vi "Make File Tree.vi"(8 "Error In":errorcluster, 10 "TreeControl in":refnum<vi>, 11 "WAD Main Cluster":T1) -> (0 "Error Out":errorcluster, 2 "TreeControl OUT":refnum<vi>, 3 "WAD Main Cluster OUT":T1)   [LabVIEW 2017]
uses:
  WAD_MainCluster.ctl
  TextureList.ctl
  PatchList.ctl
  Lumps.ctl
  <userlib>/_OpenG.lib/array/array.llb/Filter 1D Array (String)__ogtk.vi
  <vilib>/regexp/Match Regular Expression.xnode
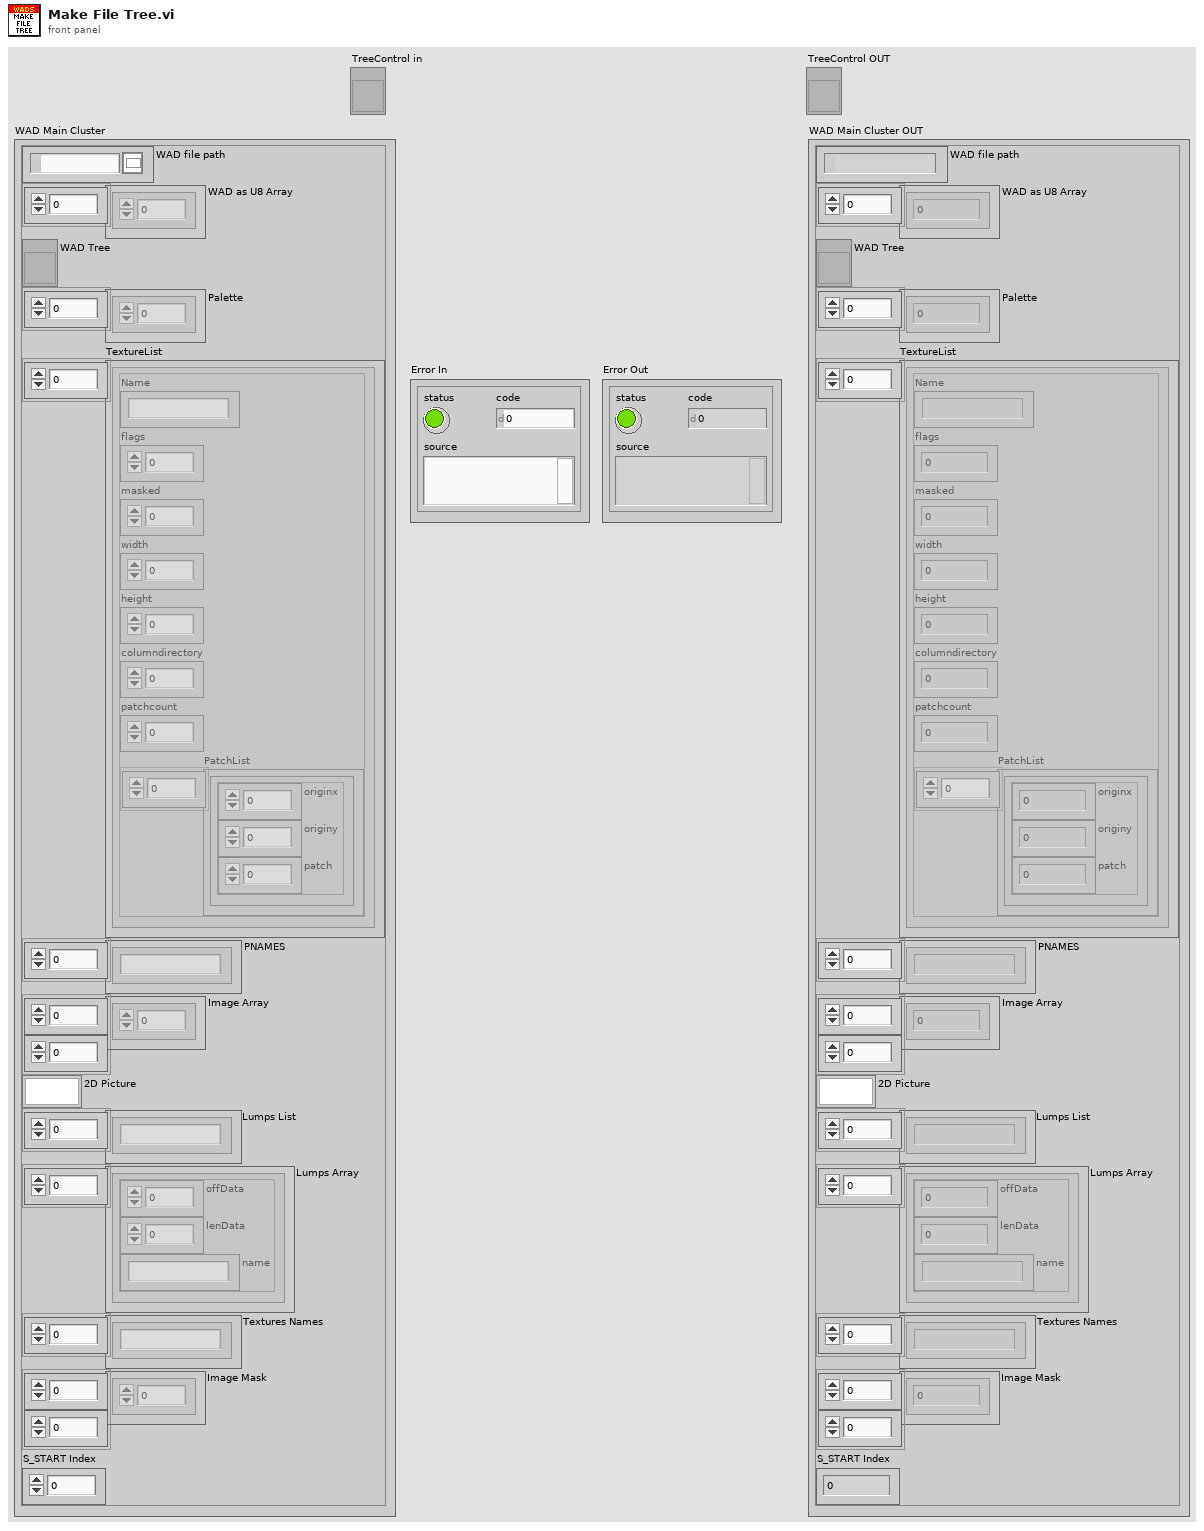
[diagram p1: front panel]
types:
  T1 = typedef "WAD_MainCluster.ctl" = cluster{"WAD file path":path, "WAD as U8 Array":u8[], "WAD Tree":refnum<vi>, "Palette":u32[], "TextureList":T2[], "PNAMES":string[], "Image Array":i16[][], "2D Picture":picture, "Lumps List":string[], "Lumps Array":T4[], "Textures Names":string[], "Image Mask":i16[][], "S_START Index":i32}
  T2 = typedef "TextureList.ctl" = cluster{"Name":string, "flags":u16, "masked":i16, "width":i16, "height":i16, "columndirectory":u32, "patchcount":i16, "PatchList":T3[]}
  T3 = typedef "PatchList.ctl" = cluster{"originx":i16, "originy":i16, "patch":i16}
  T4 = typedef "Lumps.ctl" = cluster{"offData":i32, "lenData":i32, "name":string}
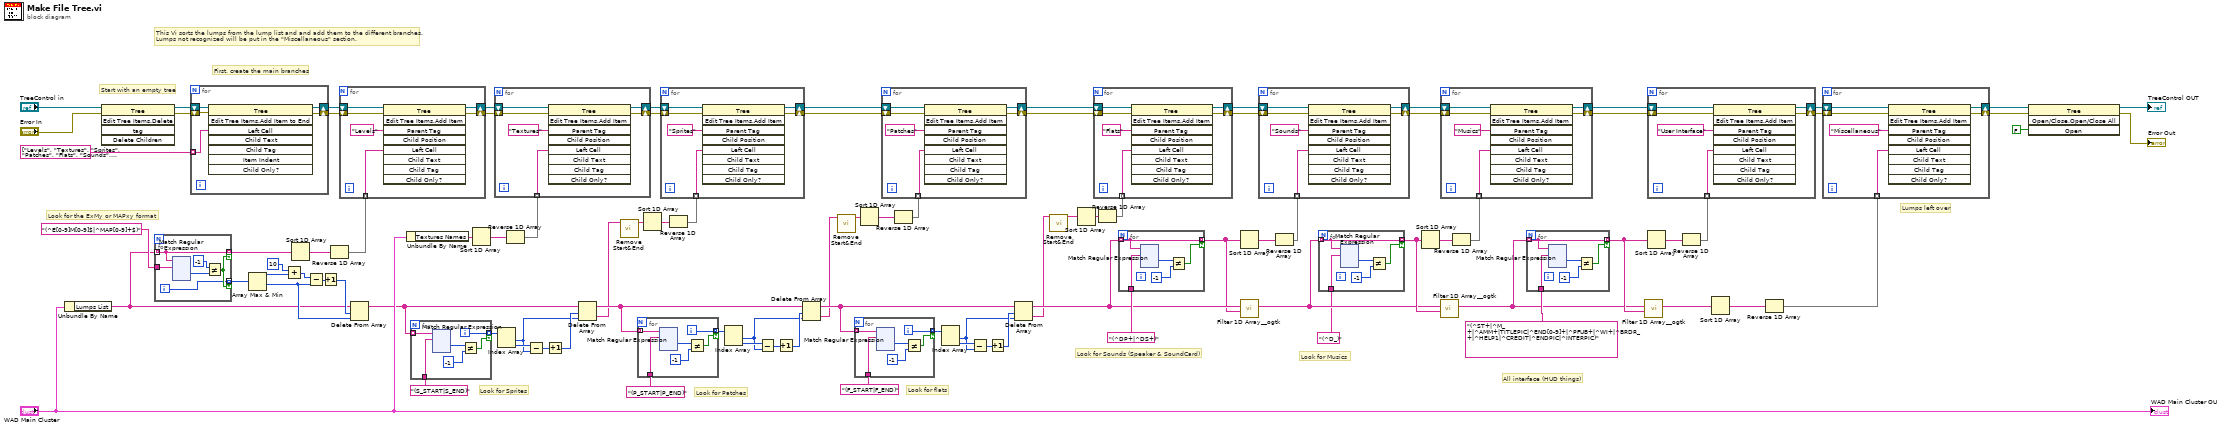
[diagram p0: block diagram]
diagram:
  # "This Vi sorts the lumps from the lump list and and add them to the different branches.\nLumps not recognized will be put in the \"Miscellaneous\" section."
  # "Start with an empty tree"
  # "First, create the main branches"
  # "Look for Musics"
  # "Lumps left over"
  # "All interface (HUD things)"
  # "Look for Sounds (Speaker & SoundCard)"
  # "Look for Sprites"
  # "Look for Patches"
  # "Look for flats"
  # "Look for the ExMy or MAPxy format"
  n1 = Unbundle By Name("WAD Main Cluster") -> ("Lumps List"=w52:string[])
  n2 = invoke on="Invoke Node" class="Tree" method="Edit Tree Items.Delete"(reference="TreeControl in", error in="Error In") -> (reference out=w88:refnum<vi>, error out=w90:errorcluster)  [unwired: 3 in, 3 out]
  n3 = for {
    tunnel: w52 -> [w99] mode=indexing
    tunnel: "(^E[0-9]M[0-9]$|^MAP[0-9]+$)" ("format string") -> [w100]
    tunnel: [w99] -> w81 mode=indexing if=w97
    tunnel: [w96] -> w62 mode=indexing if=w97
    i -> [w96]
    n4 = xnode "Match Regular Expression"("input string"=w99, "regular expression"=w100) -> ("offset past match"=w98:i32)  [unwired: 4 in, 4 out]
    n5 = Not Equal?(x=-1, y=w98) -> (x != y?=w97:bool)
  }
  n6 = for {
    tunnel: string[] ["Levels", "Textures", "Sprites", "Patches", "Flats", "Sounds", "Musics", "User Interface", "Miscellaneous"] -> [w218] mode=indexing
    shift-right: [w219] -> w91
    shift-left: w90 -> [w220]
    shift-right: [w216] -> w87
    shift-left: w88 -> [w217]
    n7 = invoke on="Invoke Node" class="Tree" method="Edit Tree Items.Add Item to End"(reference=w217, error in=w220, "Left Cell"=w218) -> (reference out=w216:refnum<vi>, error out=w219:errorcluster)  [unwired: 5 in, 6 out]
  }
  n8 = Array Max & Min(array=w62) -> (max value=w61:i32, min value=w58:i32)  [unwired: 2 out]
  n9 = Add(x=10, y=w61) -> (x+y=w59:i32)
  n10 = Sort 1D Array(array=w81) -> (sorted array=w9:string[])
  n11 = Subtract(x=w59, y=w58) -> (x-y=w57:i32)
  n12 = Increment(x=w57) -> (x+1=w56:i32)
  n13 = Reverse 1D Array(array=w9) -> (reversed array=w92:string[])
  n14 = for {
    tunnel: w92 -> [w221] mode=indexing
    shift-right: [w224] -> w27
    shift-left: w91 -> [w226]
    shift-right: [w222] -> w28
    shift-left: w87 -> [w223]
    n15 = invoke on="Invoke Node" class="Tree" method="Edit Tree Items.Add Item"(reference=w223, error in=w226, "Parent Tag"="Levels", "Left Cell"=w221) -> (reference out=w222:refnum<vi>, error out=w224:errorcluster)  [unwired: 5 in, 7 out]
  }
  n16 = Delete From Array(array=w52, length=w56, index=w58) -> (array with subset deleted=w55:string[])  [unwired: 1 out]
  n17 = Unbundle By Name("WAD Main Cluster") -> ("Textures Names"=w84:string[])
  n18 = for {
    tunnel: w55 -> [w229] mode=indexing
    tunnel: "(S_START|S_END)" ("format string") -> [w230]
    tunnel: [w227] -> w69 mode=indexing if=w228
    i -> [w227]
    n19 = xnode "Match Regular Expression"("input string"=w229, "regular expression"=w230) -> ("offset past match"=w232:i32)  [unwired: 4 in, 4 out]
    n20 = Not Equal?(x=w232, y=-1) -> (x != y?=w228:bool)
  }
  n21 = Sort 1D Array(array=w84) -> (sorted array=w8:string[])
  n22 = Index Array(array=w69) -> (element #1=w33:i32, element #2=w68:i32)  [unwired: 2 in]
  n23 = Reverse 1D Array(array=w8) -> (reversed array=w94:string[])
  n24 = for {
    shift-right: [w350] -> w25
    shift-left: w27 -> [w352]
    tunnel: w94 -> [w349] mode=indexing
    shift-right: [w347] -> w26
    shift-left: w28 -> [w348]
    n25 = invoke on="Invoke Node" class="Tree" method="Edit Tree Items.Add Item"(reference=w348, error in=w352, "Parent Tag"="Textures", "Left Cell"=w349) -> (reference out=w347:refnum<vi>, error out=w350:errorcluster)  [unwired: 5 in, 7 out]
  }
  n26 = Subtract(x=w68, y=w33) -> (x-y=w66:i32)
  n27 = Increment(x=w66) -> (x+1=w54:i32)
  n28 = Delete From Array(array=w55, length=w54, index=w33) -> (deleted portion=w22:string[], array with subset deleted=w53:string[])
  n29 = call "Remove Start&End.vi"("Lumps List"=w22) -> ("filtered array"=w21:string[])  [unwired: 10 in]
  n30 = for {
    tunnel: w53 -> [w355] mode=indexing
    tunnel: "(P_START|P_END)" ("format string") -> [w356]
    tunnel: [w353] -> w74 mode=indexing if=w354
    i -> [w353]
    n31 = xnode "Match Regular Expression"("input string"=w355, "regular expression"=w356) -> ("offset past match"=w358:i32)  [unwired: 4 in, 4 out]
    n32 = Not Equal?(x=w358, y=-1) -> (x != y?=w354:bool)
  }
  n33 = Sort 1D Array(array=w21) -> (sorted array=w7:string[])
  n34 = Reverse 1D Array(array=w7) -> (reversed array=w65:string[])
  n35 = for {
    shift-right: [w476] -> w19
    shift-left: w25 -> [w478]
    tunnel: w65 -> [w475] mode=indexing
    shift-right: [w473] -> w20
    shift-left: w26 -> [w474]
    n36 = invoke on="Invoke Node" class="Tree" method="Edit Tree Items.Add Item"(reference=w474, error in=w478, "Parent Tag"="Sprites", "Left Cell"=w475) -> (reference out=w473:refnum<vi>, error out=w476:errorcluster)  [unwired: 5 in, 7 out]
  }
  n37 = Index Array(array=w74) -> (element #1=w32:i32, element #2=w75:i32)  [unwired: 2 in]
  n38 = Subtract(x=w75, y=w32) -> (x-y=w72:i32)
  n39 = Increment(x=w72) -> (x+1=w42:i32)
  n40 = Delete From Array(array=w53, length=w42, index=w32) -> (deleted portion=w30:string[], array with subset deleted=w45:string[])
  n41 = call "Remove Start&End.vi"("Lumps List"=w30) -> ("filtered array"=w29:string[])  [unwired: 10 in]
  n42 = for {
    tunnel: w45 -> [w481] mode=indexing
    tunnel: "(F_START|F_END)" ("format string") -> [w482]
    tunnel: [w479] -> w79 mode=indexing if=w480
    i -> [w479]
    n43 = xnode "Match Regular Expression"("input string"=w481, "regular expression"=w482) -> ("offset past match"=w484:i32)  [unwired: 4 in, 4 out]
    n44 = Not Equal?(x=w484, y=-1) -> (x != y?=w480:bool)
  }
  n45 = Sort 1D Array(array=w29) -> (sorted array=w6:string[])
  n46 = Reverse 1D Array(array=w6) -> (reversed array=w71:string[])
  n47 = for {
    shift-right: [w602] -> w50
    shift-left: w19 -> [w604]
    tunnel: w71 -> [w601] mode=indexing
    shift-right: [w599] -> w51
    shift-left: w20 -> [w600]
    n48 = invoke on="Invoke Node" class="Tree" method="Edit Tree Items.Add Item"(reference=w600, error in=w604, "Parent Tag"="Patches", "Left Cell"=w601) -> (reference out=w599:refnum<vi>, error out=w602:errorcluster)  [unwired: 5 in, 7 out]
  }
  n49 = Index Array(array=w79) -> (element #1=w31:i32, element #2=w78:i32)  [unwired: 2 in]
  n50 = Subtract(x=w78, y=w31) -> (x-y=w77:i32)
  n51 = Increment(x=w77) -> (x+1=w43:i32)
  n52 = Delete From Array(array=w45, length=w43, index=w31) -> (deleted portion=w24:string[], array with subset deleted=w36:string[])
  n53 = call "Remove Start&End.vi"("Lumps List"=w24) -> ("filtered array"=w23:string[])  [unwired: 10 in]
  n54 = Sort 1D Array(array=w23) -> (sorted array=w5:string[])
  n55 = Reverse 1D Array(array=w5) -> (reversed array=w76:string[])
  n56 = for {
    shift-right: [w608] -> w48
    shift-left: w50 -> [w610]
    tunnel: w76 -> [w607] mode=indexing
    shift-right: [w605] -> w49
    shift-left: w51 -> [w606]
    n57 = invoke on="Invoke Node" class="Tree" method="Edit Tree Items.Add Item"(reference=w606, error in=w610, "Parent Tag"="Flats", "Left Cell"=w607) -> (reference out=w605:refnum<vi>, error out=w608:errorcluster)  [unwired: 5 in, 7 out]
  }
  n58 = for {
    tunnel: w36 -> [w612] mode=indexing
    tunnel: "(^DP+|^DS+)" ("format string") -> [w613]
    tunnel: [w612] -> w35 mode=indexing if=w611
    n59 = xnode "Match Regular Expression"("input string"=w612, "regular expression"=w613) -> ("offset past match"=w615:i32)  [unwired: 4 in, 4 out]
    n60 = Not Equal?(x=w615, y=-1) -> (x != y?=w611:bool)
  }
  n61 = call-poly <userlib>:"Filter 1D Array__ogtk.vi"("items to filter"=w35, "array"=w36) -> ("filtered array"=w17:string[])  [unwired: 4 in, 1 out]
  n62 = Sort 1D Array(array=w35) -> (sorted array=w4:string[])
  n63 = Reverse 1D Array(array=w4) -> (reversed array=w63:string[])
  n64 = for {
    shift-right: [w733] -> w14
    shift-left: w48 -> [w735]
    tunnel: w63 -> [w732] mode=indexing
    shift-right: [w730] -> w15
    shift-left: w49 -> [w731]
    n65 = invoke on="Invoke Node" class="Tree" method="Edit Tree Items.Add Item"(reference=w731, error in=w735, "Parent Tag"="Sounds", "Left Cell"=w732) -> (reference out=w730:refnum<vi>, error out=w733:errorcluster)  [unwired: 5 in, 7 out]
  }
  n66 = for {
    tunnel: w17 -> [w737] mode=indexing
    tunnel: "(^D_)" ("format string") -> [w738]
    tunnel: [w737] -> w18 mode=indexing if=w736
    n67 = xnode "Match Regular Expression"("input string"=w737, "regular expression"=w738) -> ("offset past match"=w740:i32)  [unwired: 4 in, 4 out]
    n68 = Not Equal?(x=w740, y=-1) -> (x != y?=w736:bool)
  }
  n69 = Sort 1D Array(array=w18) -> (sorted array=w3:string[])
  n70 = call-poly <userlib>:"Filter 1D Array__ogtk.vi"("items to filter"=w18, "array"=w17) -> ("filtered array"=w10:string[])  [unwired: 4 in, 1 out]
  n71 = Reverse 1D Array(array=w3) -> (reversed array=w11:string[])
  n72 = for {
    shift-right: [w858] -> w12
    shift-left: w14 -> [w860]
    tunnel: w11 -> [w857] mode=indexing
    shift-right: [w855] -> w13
    shift-left: w15 -> [w856]
    n73 = invoke on="Invoke Node" class="Tree" method="Edit Tree Items.Add Item"(reference=w856, error in=w860, "Parent Tag"="Musics", "Left Cell"=w857) -> (reference out=w855:refnum<vi>, error out=w858:errorcluster)  [unwired: 5 in, 7 out]
  }
  n74 = for {
    tunnel: w10 -> [w862] mode=indexing
    tunnel: "(^ST+|^M_+|^AMM+|TITLEPIC|^END[0-9]+|^PFUB+|^WI+|^BRDR_+|^HELP1|^CREDIT|^ENDPIC|^INTERPIC)" ("format string") -> [w863]
    tunnel: [w862] -> w34 mode=indexing if=w861
    n75 = xnode "Match Regular Expression"("input string"=w862, "regular expression"=w863) -> ("offset past match"=w865:i32)  [unwired: 4 in, 4 out]
    n76 = Not Equal?(x=w865, y=-1) -> (x != y?=w861:bool)
  }
  n77 = call-poly <userlib>:"Filter 1D Array__ogtk.vi"("items to filter"=w34, "array"=w10) -> ("filtered array"=w38:string[])  [unwired: 4 in, 1 out]
  n78 = Sort 1D Array(array=w34) -> (sorted array=w1:string[])
  n79 = Reverse 1D Array(array=w1) -> (reversed array=w37:string[])
  n80 = for {
    shift-right: [w983] -> w41
    shift-left: w12 -> [w985]
    tunnel: w37 -> [w982] mode=indexing
    shift-right: [w980] -> w40
    shift-left: w13 -> [w981]
    n81 = invoke on="Invoke Node" class="Tree" method="Edit Tree Items.Add Item"(reference=w981, error in=w985, "Parent Tag"="User Interface", "Left Cell"=w982) -> (reference out=w980:refnum<vi>, error out=w983:errorcluster)  [unwired: 5 in, 7 out]
  }
  n82 = Sort 1D Array(array=w38) -> (sorted array=w2:string[])
  n83 = Reverse 1D Array(array=w2) -> (reversed array=w44:string[])
  n84 = for {
    shift-right: [w989] -> w46
    shift-left: w41 -> [w991]
    tunnel: w44 -> [w988] mode=indexing
    shift-right: [w986] -> w47
    shift-left: w40 -> [w987]
    n85 = invoke on="Invoke Node" class="Tree" method="Edit Tree Items.Add Item"(reference=w987, error in=w991, "Parent Tag"="Miscellaneous", "Left Cell"=w988) -> (reference out=w986:refnum<vi>, error out=w989:errorcluster)  [unwired: 5 in, 7 out]
  }
  n86 = invoke on="Invoke Node" class="Tree" method="Open/Close.Open/Close All"(reference=w47, error in=w46, "Open"=FALSE ("Open?")) -> (reference out=→"TreeControl OUT":refnum<vi>, error out=→"Error Out":errorcluster)  [unwired: 1 in, 2 out]
  "WAD Main Cluster OUT" <- "WAD Main Cluster"
